vi "Unsubscribe (async).vi"(8 "error in (no error)":errorcluster, 10 "Topic":string, 11 "WAMP Client in":refnum<class "WAMP Client.lvclass">) -> (0 "error out":errorcluster, 2 "Result notifier":refnum<notifier>, 3 "WAMP Client out":refnum<class "WAMP Client.lvclass">)   [LabVIEW 2020, in "wamplv.lvlib" / "WAMP Client.lvclass"]
uses:
  WAMP Client.lvclass
  TypeDef/UNSUBSCRIBE Result.ctl
  API/TypeDefs/Combined error.ctl
  API/TypeDefs/WAMP error.ctl
  TypeDef/UNSUBSCRIBE Request Data.ctl
  TypeDef/Internal Message Type.ctl
  WAMP Client.lvclass/WAMP Client.ctl
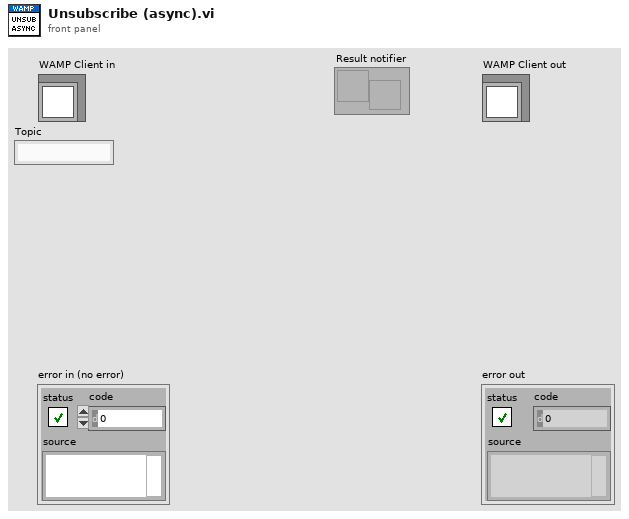
[diagram p1: front panel]
types:
  T1 = typedef "wamplv.lvlib/WAMP Client.lvclass/Internal Message Type.ctl" = enum16{"Subscribe", "Handle Subscribed", "Handle Event", "Unsubscribe", "Handle Unsubscribed", "Publish", "Handled Published", "Goodbye", "Handle Goodbye", "Call", "Handle Result", "Register", "Handle Registered", "Unregister", "Handle Unregistered", "Handle Invocation", "Yield", "Error"}
  T2 = typedef "wamplv.lvlib/WAMP Client.lvclass/UNSUBSCRIBE Request Data.ctl" = cluster{"Topic":string, "Unsubscrube result notifier":refnum<notifier>}
  T3 = typedef "wamplv.lvlib/WAMP Client.lvclass/UNSUBSCRIBE Result.ctl" = cluster{"Success?":bool, "Combined Error":T4}
  T4 = typedef "wamplv.lvlib/WAMP Client.lvclass/Combined error.ctl" = cluster{"Error?":bool, "WAMP Error":T5, "Error":errorcluster}
  T5 = typedef "wamplv.lvlib/WAMP Client.lvclass/WAMP error.ctl" = cluster{"Details":string, "ArgumentKw Payload":string, "Error?":bool, "Error URI":string, "Arguments Payload":string}
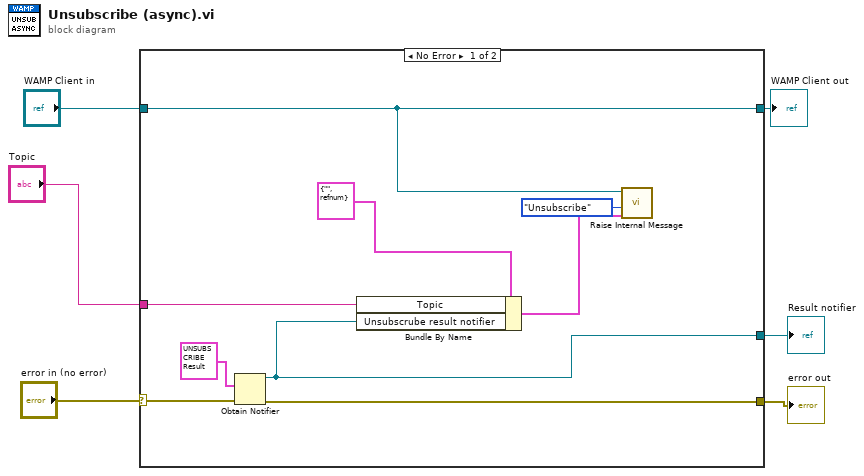
[diagram p0: block diagram]
diagram:
  n1 = case shown="No Error" "error in (no error)" {
    selector: "error in (no error)" -> [w10 w17]
    tunnel: [w9 w17] -> w5
    tunnel: [w15 w16] -> w3
    tunnel: "WAMP Client in" -> [w15 w16]
    tunnel: "Topic" -> [w13 _]
    tunnel: [w7 _] -> w1
    frame No Error {
      n2 = Obtain Notifier(notification data type=T3 {"Success?"=FALSE, "Combined Error"={"Error?"=FALSE, "WAMP Error"={"Details"="", "ArgumentKw Payload"="{}", "Error?"=FALSE, "Error URI"="", "Arguments Payload"=""}, "Error"={"status"=FALSE, "code"=0, "source"=""}}} ("Subcsribe Result"), error in (no error)=w10) -> (notifier out=w7:refnum<notifier>, error out=w9:errorcluster)  [unwired: 2 in, 1 out]
      n3 = Bundle By Name(cluster=T2 {"Topic"="", "Unsubscrube result notifier"=refnum} ("Cluster"), "Topic"=w13, "Unsubscrube result notifier"=w7) -> (w14:T2)
      n4 = call "Raise Internal Message.vi"("Variant"=w14, "Internal Message Type"=Internal_Message_Type."Unsubscribe", "WAMP Client in"=w15) -> ()  [unwired: 7 in, 2 out]
    }
    frame Error {
    }
  }
  "error out" <- w5
  "WAMP Client out" <- w3
  "Result notifier" <- w1
